vi "change data.vi"(0 "register in":T1, 1 "task in":T2={"Task Info"={"Accele Task"=[], "Simulate"=FALSE, "采样率"={"AISampleRate"=10123, "CouplingType"=10000, "Butter"=1000}, "Trig"={"PreTrigCNT"=0, "TriggerMode"=enum."中间触发", "TriggerSource"=enum."软件触发", "ATRTriggerChannel"=enum."通道0", "TriggerDir"=enum."下降沿触发", "TrigLevelVolt"=0.0, "bAvailableTrig"=FALSE}, "clock"={"EN"=FALSE, "clocksource"=enum."内部时钟", "outclocksource"=enum."Trig0"}, "delay(S)"=0.0}, "datain"={"nSegmentCount"=0, "chaneldataSize"=8192, "t0 in"=timestamp(0 s since 1904-01-01), "nsegmentsize"=0, "chanelcouter"=0}, "times"=0.0, "timer"=[], "\nen"=FALSE} {"Task Info"."采样率"."CouplingType" items=["直流耦合", "交流耦合"]}, 2 "buffer":u16[](array[numeric]), 3 "error in":errorcluster, 4 "Temperature":sgl format="%0.6f") -> (7 "register out":T1, 8 "task out":T2={"Task Info"={"Accele Task"=[], "Simulate"=FALSE, "采样率"={"AISampleRate"=10123, "CouplingType"=10000, "Butter"=1000}, "Trig"={"PreTrigCNT"=0, "TriggerMode"=enum."中间触发", "TriggerSource"=enum."软件触发", "ATRTriggerChannel"=enum."通道0", "TriggerDir"=enum."下降沿触发", "TrigLevelVolt"=0.0, "bAvailableTrig"=FALSE}, "clock"={"EN"=FALSE, "clocksource"=enum."内部时钟", "outclocksource"=enum."Trig0"}, "delay(S)"=0.0}, "datain"={"nSegmentCount"=0, "chaneldataSize"=8192, "t0 in"=timestamp(0 s since 1904-01-01), "nsegmentsize"=0, "chanelcouter"=0}, "times"=0.0, "timer"=[], "\nen"=FALSE} {"Task Info"."采样率"."CouplingType" items=["直流耦合", "交流耦合"]}, 9 "data":waveform(dbl)[](array[waveform]), 10 "error out":errorcluster)   [LabVIEW 2009]
uses:
  PCI8532_32.dll
  Ctrls/Acceleration Channel Config_Ctrls-某型振动实验台测试系统.ctl
  Ctrls/Sample Information.ctl
  Ctrls/Trig.ctl
  Ctrls/clock.ctl
  Ctrls/Task Info.ctl
  Ctrls/DATA info.ctl
  Ctrls/task.ctl
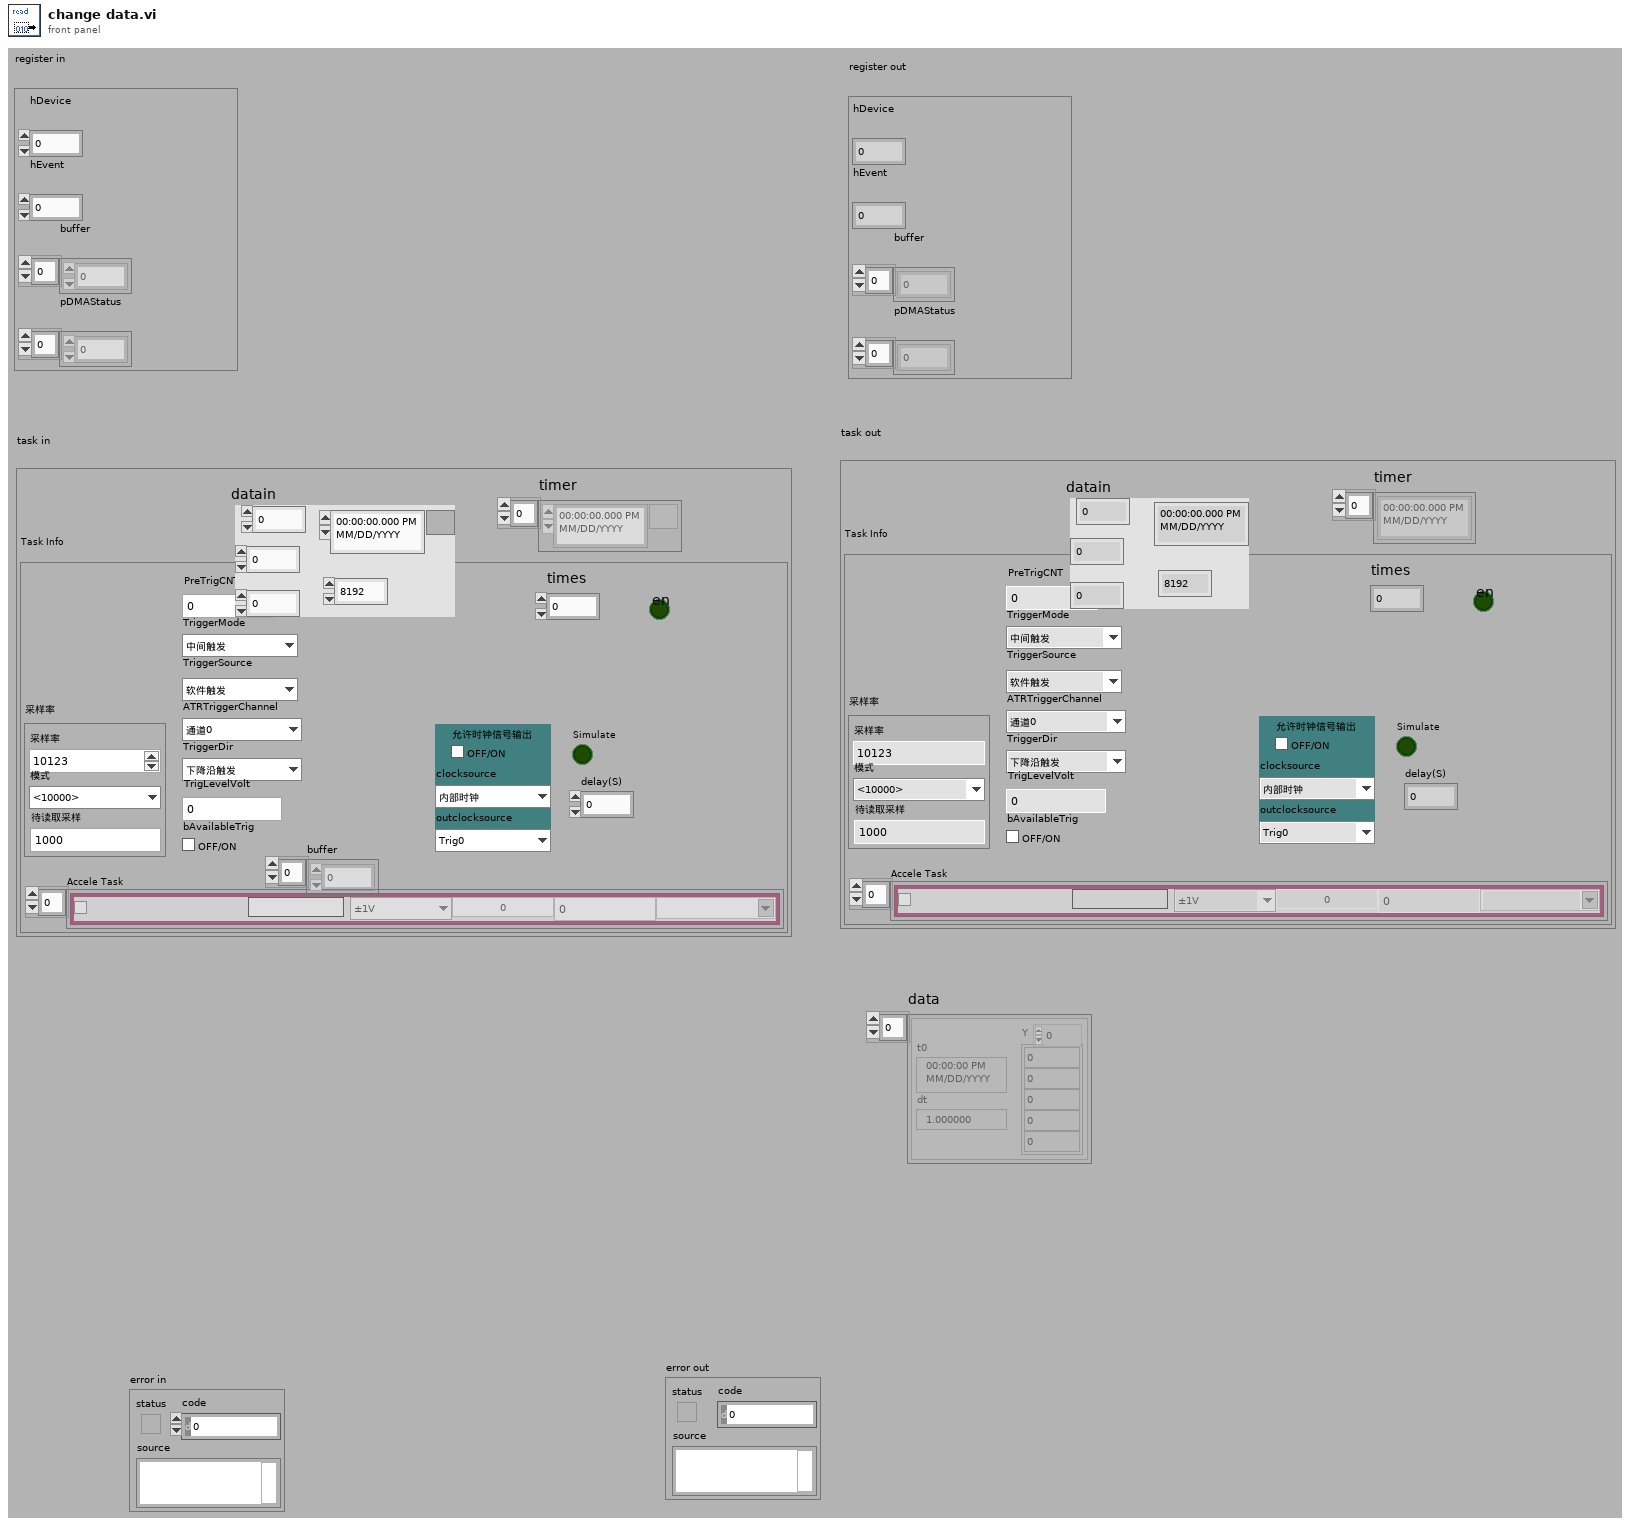
[diagram p1: front panel]
types:
  T1 = cluster{"hDevice":i32, "hEvent":i32, "buffer":u16[], "pDMAStatus":i32[]}
  T2 = typedef "task.ctl" = cluster{"Task Info":T3, "datain":T8, "times":dbl, "timer":timestamp[], "\nen":bool}
  T3 = typedef "Task Info.ctl" = cluster{"Accele Task":T4[], "Simulate":bool, "采样率":T5, "Trig":T6, "clock":T7, "delay(S)":dbl}
  T4 = typedef "Acceleration Channel Config_Ctrls-某型振动实验台测试系统.ctl" = cluster{"Enable":bool, "Name":string, "range":enum16{"±1V", "±5V"}, "SensValue":dbl, "PhysicalName":string, "off":dbl, "Sensunits":string}
  T5 = typedef "Sample Information.ctl" = cluster{"AISampleRate":i32, "CouplingType":i32, "Butter":i32}
  T6 = typedef "Trig.ctl" = cluster{"PreTrigCNT":i32, "TriggerMode":enum16{"中间触发", "后触发", "预触发", "硬件延时触发"}, "TriggerSource":enum16{"软件触发", "DTR信号源", "ATR信号源", "Triger信号触发"}, "ATRTriggerChannel":enum16{"通道0", "通道1", "通道2", "通道3"}, "TriggerDir":enum16{"下降沿触发", "上升沿触发", "上下边没均触发"}, "TrigLevelVolt":sgl, "bAvailableTrig":bool}
  T7 = typedef "clock.ctl" = cluster{"EN":bool, "clocksource":enum16{"内部时钟", "外部时钟"}, "outclocksource":enum16{"Trig0", "Trig1", "Trig2", "Trig3", "Trig4", "Trig5", "Trig6", "Trig7", "PXI_STAR"}}
  T8 = typedef "DATA info.ctl" = cluster{"nSegmentCount":i32, "chaneldataSize":i32, "t0 in":timestamp, "nsegmentsize":i32, "chanelcouter":i32}
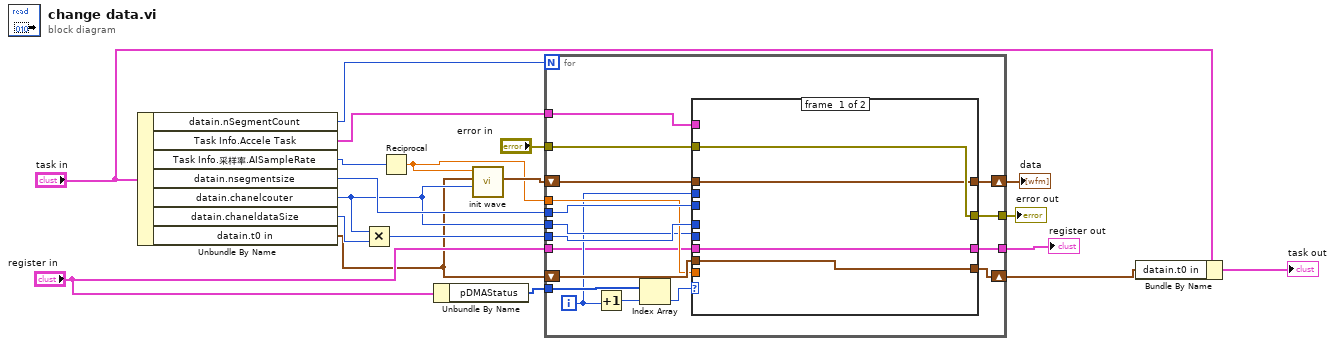
[diagram p0: block diagram]
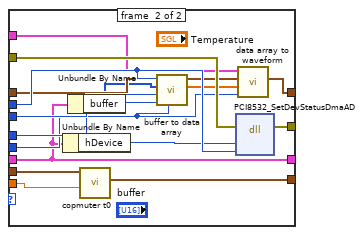
[diagram p2: hidden frame]
diagram:
  n1 = Unbundle By Name("task in") -> ("datain.nSegmentCount"=w14:i32, "Task Info.Accele Task"=w17:T4[], "Task Info.采样率.AISampleRate"=w16:i32, "datain.nsegmentsize"=w12:i32, "datain.chanelcouter"=w8:i32, "datain.chaneldataSize"=w11:i32, "datain.t0 in"=w2:timestamp)
  n2 = Multiply(x=w8, y=w11) -> (x*y=w18:i32)
  n3 = Reciprocal(x=w16) -> (1/x=w9:dbl)
  n4 = Unbundle By Name("register in") -> ("pDMAStatus"=w6:i32[])
  n5 = call "init wave.vi"("chanelcouter"=w8, "t0"=w2, "dt"=w9) -> ("initialized array"=w10:waveform(dbl)[])  [unwired: 8 out]
  n6 = for {
    N: w14 -> [_]
    tunnel: w6 -> [w36]
    tunnel: "error in" -> [w34]
    tunnel: [w33] -> w1
    tunnel: w12 -> [w32]
    tunnel: w18 -> [w31]
    tunnel: w17 -> [w30]
    shift-right: [w27] -> w15
    shift-left: w2 -> [w29]
    tunnel: w9 -> [w28]
    tunnel: w8 -> [w26]
    shift-right: [w25] -> w13
    shift-left: w10 -> [w24]
    tunnel: "register in" -> [w21]
    tunnel: [w20] -> w3
    i -> [w23]
    n7 = Increment(x=w23) -> (x+1=w22:i32)
    n8 = Index Array(array=w36, index=w22) -> (element=w35:i32)
    n9 = case shown="1" w35 {
      tunnel: w23 -> [_ w51]
      tunnel: w34 -> [w40 w56]
      tunnel: [w40 w55] -> w33
      tunnel: w32 -> [_ w50]
      tunnel: w31 -> [_ w49]
      tunnel: w26 -> [_ w44]
      tunnel: w30 -> [_ w48]
      tunnel: w29 -> [w39 w54]
      tunnel: w28 -> [_ w53]
      tunnel: [w39 w52] -> w27
      tunnel: [w38 w45] -> w25
      tunnel: w24 -> [w38 w47]
      tunnel: w21 -> [w37 w42]
      tunnel: [w37 w42] -> w20
      frame #0 {
      }
      frame #1 {
        n10 = Unbundle By Name(w42) -> ("hDevice"=w43:i32)
        n11 = Unbundle By Name(w42) -> ("buffer"=w41:u16[])
        n12 = call "copmuter t0.vi"("time"=w53, "t0 in"=w54) -> ("t0 out"=w52:timestamp)  [unwired: 2 in, 7 out]
        n13 = call "buffer to data array.vi"(6:w44, "set para 2"=w49, 9:w50, "buffer"=w41, "i"=w51) -> ("data"=w46:dbl[])  [unwired: 6 out]
        n14 = dll-call lib="PCI8532_32.dll" fn="PCI8532_SetDevStatusDmaAD" ("SetDevStatusDmaAD")(error in=w56, "hDevice"=w43, "iClrBufferID"=w51) -> (error out=w55:errorcluster)  [unwired: 4 in, 2 out]
        n15 = call "data array to waveform.vi"(8:w44, "Main Vari"=w46, 10:w47, "data"=w48) -> ("wave out"=w45:waveform(dbl)[])  [unwired: 1 in, 6 out]
      }
    }
  }
  "data" <- w13
  "register out" <- w3
  "error out" <- w1
  n16 = Bundle By Name(cluster="task in", "datain.t0 in"=w15) -> (→"task out":T2)
